vi "low_cap.vi"(11 "num":dbl) -> (3 "lim":dbl)   [LabVIEW 2011]
panel:
  # "Caps numbers to (0,1)"
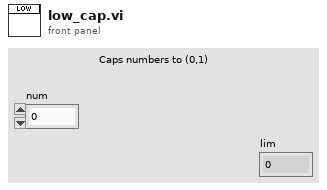
[diagram p1: front panel]
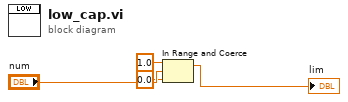
[diagram p0: block diagram]
diagram:
  n1 = In Range and Coerce(upper limit=1.0, x="num", lower limit=0.0) -> (coerced(x)=→"lim":dbl)  [unwired: 1 out]
